vi "Fuzzy_PT100_V2.vi"() -> ()   [LabVIEW 2025]
uses:
  <vilib>/DAQmx/write.llb/DAQmx Write (Digital 1D Bool 1Chan 1Samp).vi
  <vilib>/addons/Fuzzy Logic/FL Fuzzy Controller (SISO).vi
  <vilib>/DAQmx/create/channels.llb/DAQmx Create Channel (DO-Digital Output).vi
  <vilib>/DAQmx/miscellaneous.llb/DAQmx Fill In Error Info.vi
  <vilib>/addons/Fuzzy Logic/NI_Fuzzy_Logic_API.lvlib
  <resource>/objmgr/daqmx.rc
panel:
  in  "stop 3":bool
  out "Low Time":dbl
  out "High Yime":dbl
  in  "Digital Lines":tag
  in  "stop 2":bool
  out "Waveform Chart":dynamicdata(graph)
  out "Duty":dbl
  out "Error":dbl
  in  "Set point":dbl
  out "Temp":dbl
  in  "file path":path
  out "data":dbl
  in  "stop":bool
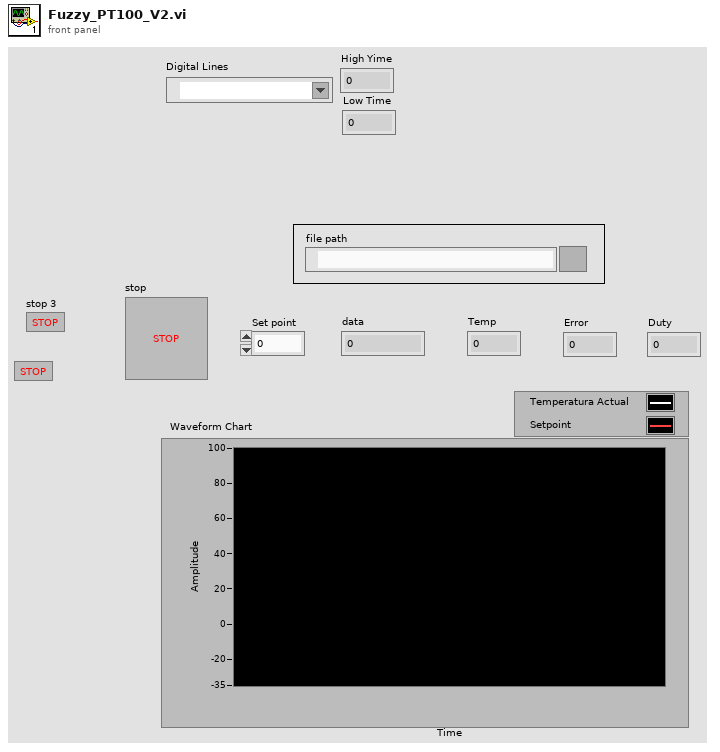
[diagram p1: front panel]
types:
  T1 = typedef "NI_Fuzzy_Logic_API.lvlib/FL System.ctl" = cluster{"input variables":T2[], "output variables":T2[], "rules":T5[], "defuzzification method":T11, "description":string, "user MF interpolating polynomials":T12[]}
  T2 = typedef "NI_Fuzzy_Logic_API.lvlib/FL Variable.ctl" = cluster{"name":string, "range":dbl[], "MFs":T3[]}
  T3 = typedef "NI_Fuzzy_Logic_API.lvlib/FL Membership Function.ctl" = cluster{"name":string, "shape":T4, "points":dbl[], "color":u32, "user-defined shape index":i32}
  T4 = typedef "NI_Fuzzy_Logic_API.lvlib/FL Membership Function Shape.ctl" = u16
  T5 = typedef "NI_Fuzzy_Logic_API.lvlib/FL Rule.ctl" = cluster{"antecedents":T6[], "antecedent connective":T8, "consequents":T9[], "consequent implication":T10, "degree of support":dbl}
  T6 = typedef "NI_Fuzzy_Logic_API.lvlib/FL Antecedent.ctl" = cluster{"Var Index":i32, "MF Index":i32, "Cond":T7}
  T7 = typedef "NI_Fuzzy_Logic_API.lvlib/FL Modifier.ctl" = u16
  T8 = typedef "NI_Fuzzy_Logic_API.lvlib/FL Antecedent Connective.ctl" = u16
  T9 = typedef "NI_Fuzzy_Logic_API.lvlib/FL Consequent.ctl" = cluster{"Var Index":i32, "MF Index":i32, "Cond":T7}
  T10 = typedef "NI_Fuzzy_Logic_API.lvlib/FL Consequent Implication.ctl" = u16
  T11 = typedef "NI_Fuzzy_Logic_API.lvlib/FL Defuzzification.ctl" = u16
  T12 = typedef "NI_Fuzzy_Logic_API.lvlib/FL Interpolating polynomials.ctl" = cluster{"X":dbl[], "Y":dbl[], "Y(x) coeff":dbl[][], "X(y) coeff":dbl[][], "Area(y) coeff":dbl[][], "coa_x(y) coeff":dbl[][]}
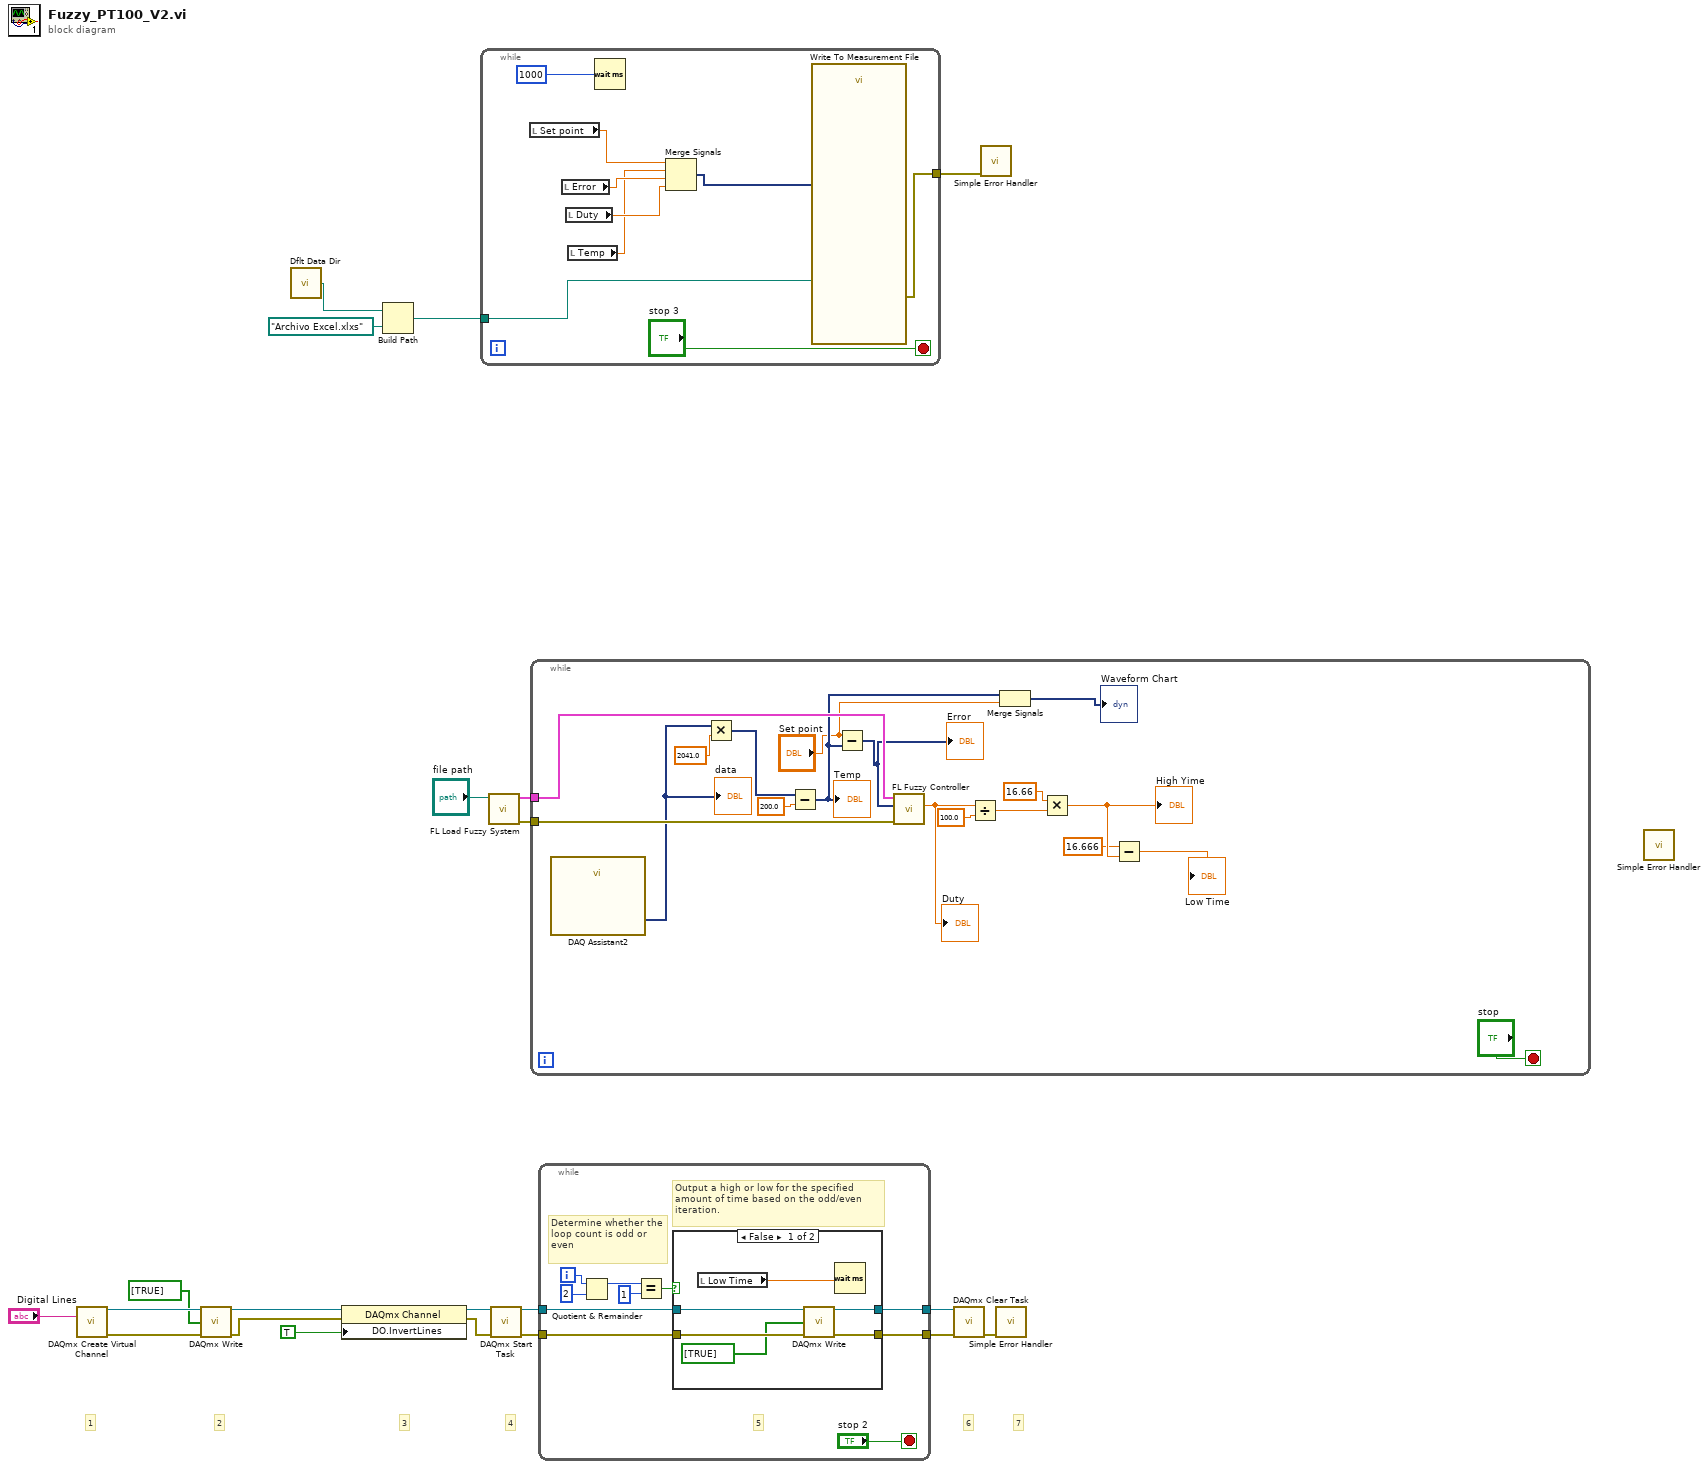
[diagram p0: block diagram]
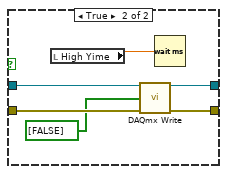
[diagram p2: hidden frame]
diagram:
  # "7"
  # "6"
  # "4"
  # "3"
  # "2"
  # "1"
  n1 = call-poly <vilib>:"DAQmx Create Virtual Channel.vi"("lines"="Digital Lines") -> ("task out"=w18:refnum<k21>, "error out"=w17:errorcluster)  [unwired: 13 in]
  n2 = call-poly <vilib>:"DAQmx Write.vi"("task/channels in"=w18, "data"=bool[] [TRUE], "error in"=w17) -> ("task out"=w9:refnum<k21>, "error out"=w5:errorcluster)  [unwired: 10 in, 1 out]
  n3 = call <vilib>:"Dflt Data Dir.vi"() -> ("App:Default Data Directory"=w3:path)
  n4 = property class="DAQmx Channel"(reference=w9, error in=w5, "DO.InvertLines"=TRUE) -> (reference out=w8:refnum<k21>, error out=w7:errorcluster)
  n5 = Build Path(base path=w3, name or relative path=path "Archivo Excel.xlxs") -> (appended path=w2:path)
  n6 = while {
    tunnel: w2 -> [w29]
    tunnel: [w28] -> w1
    stop <- "stop 3" stop-if-true
    n7 = local read "Set point"() -> (w24:dbl)
    n8 = local read "Error"() -> (w26:dbl)
    n9 = local read "Duty"() -> (w23:dbl)
    n10 = local read "Temp"() -> (w22:dbl)
    n11 = Wait (ms)(milliseconds to wait=u32 1000) -> ()  [unwired: 1 out]
    n12 = Merge Signals(w24, w22, w26, w23) -> (w25:dynamicdata)
    n13 = call "Write To Measurement File"("Signals"=w25, "Filename"=w29) -> ("error out"=w28:errorcluster)  [unwired: 15 in, 2 out]
  }
  n14 = call <vilib>:"FL Load Fuzzy System.vi"("file path"="file path") -> ("error out"=w19:errorcluster, "fuzzy system out"=w20:T1)  [unwired: 9 in]
  n15 = call <vilib>:"DAQmx Start Task.vi"("task/channels in"=w8, "error in"=w7) -> ("task out"=w16:refnum<k21>, "error out"=w15:errorcluster)  [unwired: 12 in]
  n16 = while {
    tunnel: w20 -> [w47]
    tunnel: w19 -> [w46]
    stop <- "stop" stop-if-true
    n17 = call "DAQ Assistant2"() -> ("data"=w45:dynamicdata)  [unwired: 17 in, 2 out]
    "data" <- w45
    n18 = Multiply(x=w45, y=2041.0) -> (x*y=w42:dynamicdata)
    n19 = Subtract(x=w42, y=200.0) -> (x-y=w32:dynamicdata)
    "Temp" <- w32
    n20 = Subtract(x="Set point", y=w32) -> (x-y=w33:dynamicdata)
    "Error" <- w33
    n21 = call-poly <vilib>:"FL Fuzzy Controller.vi"("error in (no error)"=w46, "input value"=w33, "fuzzy system in"=w47) -> ("output value"=w37:dbl)  [unwired: 4 in, 4 out]
    "Duty" <- w37
    n22 = Divide(x=w37, y=100.0) -> (x/y=w39:dbl)
    n23 = Merge Signals(w32, "Set point") -> (→"Waveform Chart":dynamicdata)
    n24 = Multiply(x=16.66 ("y"), y=w39) -> (x*y=w36:dbl)
    "High Yime" <- w36
    n25 = Subtract(x=16.666, y=w36) -> (x-y=→"Low Time":dbl)
  }
  n26 = while {
    tunnel: w16 -> [w58]
    tunnel: w15 -> [w57]
    tunnel: [w56] -> w14
    tunnel: [w55] -> w13
    i -> [w53]
    stop <- "stop 2" stop-if-true
    # "5"
    # "Output a high or low for the specified\namount of time based on the odd/even\niteration."
    # "Determine whether the loop count is odd or even"
    n27 = Quotient & Remainder(x=w53, y=2) -> (x-y*floor(x/y)=w51:i32)  [unwired: 1 out]
    n28 = Equal?(x=w51, y=1) -> (x = y?=w49:bool)
    n29 = case shown="False" w49 {
      tunnel: w58 -> [w62 w70]
      tunnel: w57 -> [w61 w69]
      tunnel: [w63 w68] -> w56
      tunnel: [w64 w67] -> w55
      frame False {
        n30 = local read "Low Time"() -> (w59:dbl)
        n31 = call-poly <vilib>:"DAQmx Write.vi"("task/channels in"=w62, "data"=bool[] [TRUE], "error in"=w61) -> ("task out"=w64:refnum<k21>, "error out"=w63:errorcluster)  [unwired: 10 in, 1 out]
        n32 = Wait (ms)(milliseconds to wait=w59) -> ()  [unwired: 1 out]
      }
      frame True {
        n33 = local read "High Yime"() -> (w65:dbl)
        n34 = call-poly <vilib>:"DAQmx Write.vi"("task/channels in"=w70, "data"=bool[] [FALSE], "error in"=w69) -> ("task out"=w67:refnum<k21>, "error out"=w68:errorcluster)  [unwired: 10 in, 1 out]
        n35 = Wait (ms)(milliseconds to wait=w65) -> ()  [unwired: 1 out]
      }
    }
  }
  n36 = call <vilib>:"DAQmx Clear Task.vi"("task in"=w13, "error in"=w14) -> ("error out"=w12:errorcluster)  [unwired: 13 in]
  n37 = call <vilib>:"Simple Error Handler.vi"("error in (no error)"=w1) -> ()  [unwired: 4 in, 5 out]
  n38 = call <vilib>:"Simple Error Handler.vi"("error in (no error)"=w12) -> ()  [unwired: 4 in, 5 out]
  n39 = call <vilib>:"Simple Error Handler.vi"() -> ()  [unwired: 5 in, 5 out]
